vi "Snap.vi"(8 "error in (no error)":errorcluster, 11 "MQTT-Server in":refnum<class "MQTT-Server.lvclass">) -> (0 "error out":errorcluster, 3 "MQTT-Server out":refnum<class "MQTT-Server.lvclass">)   [LabVIEW 2023]
uses:
  MQTT-Server.lvclass
  MQTT-Server.lvclass/MQTT-Server.ctl
  C:/Program Files/National Instruments/LabVIEW 2023/vi.lib/ActorFramework/Actor/Actor.lvclass
  C:/Users/KIV4BP/Documents/Projects/mqtt-budlug/source/MQTT-Server/MQTT-Server/MQTT-Server.lvclass
panel:
  out "Chart":waveform(dbl)[](graph)
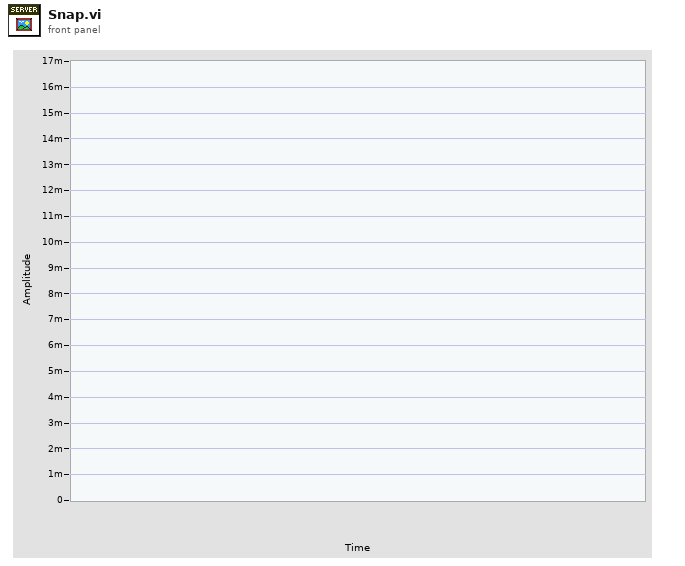
[diagram p1: front panel]
types:
  T1 = typedef "imagedata.ctl" = cluster{"image type":i32, "image depth":i32, "image":u8[], "mask":u8[], "colors":u32[], "Rectangle":cluster{"left":i16, "top":i16, "right":i16, "bottom":i16}}
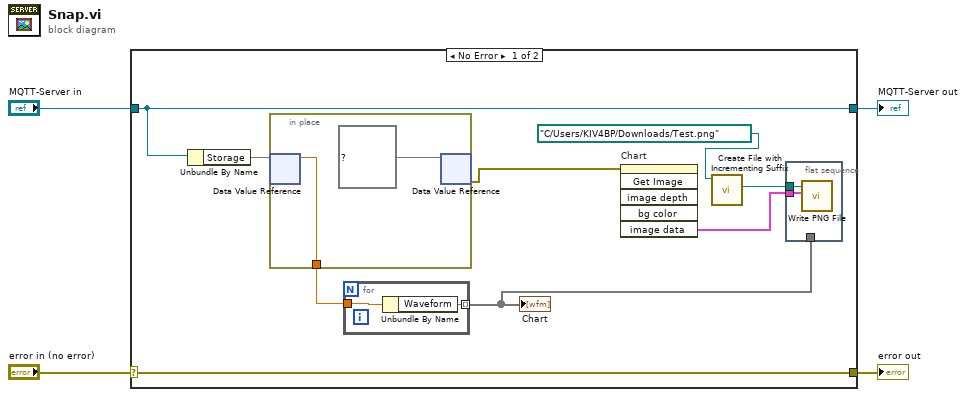
[diagram p0: block diagram]
diagram:
  n1 = case shown="No Error" "error in (no error)" {
    selector: "error in (no error)" -> [w13 w21]
    tunnel: [w13 w21] -> w3
    tunnel: [w12 w20] -> w1
    tunnel: "MQTT-Server in" -> [w12 w20]
    frame No Error {
      n2 = Unbundle By Name(w12) -> ("Storage"=w11)
      n3 = in-place {
        in-place-border: [w18] -> w10
        n4 = in-place-dvr #1(w11) -> (w18:dbl)  [unwired: 1 out]
        n5 = in-place-dvr #1(map{string, waveform(dbl)} {} ("data value")) -> (w8:errorcluster)  [unwired: 1 out]
      }
      n6 = for {
        tunnel: w10 -> [w17]
        tunnel: [w16] -> w5 mode=indexing
        n7 = Unbundle By Name(w17) -> ("Waveform"=w16)
      }
      "Chart" <- w5
      n8 = invoke on="Chart" class="WFChart (strict)" method="Get Image"(error in=w8) -> ("image data"=w9:T1)  [unwired: 5 in, 5 out]
      n9 = call <vilib>:"Create File with Incrementing Suffix.vi"("file path"=path "C:/Users/KIV4BP/Downloads/Test.png" ("path to PNG file")) -> ("actual path"=w6:path)  [unwired: 8 in, 2 out]
      n10 = flat-sequence {
        tunnel: w9 -> [w15]
        tunnel: w6 -> [w14]
        tunnel: w5 -> [_]
        frame #0 {
          n11 = call <vilib>:"Write PNG File.vi"("image data"=w15, "path to PNG file"=w14) -> ()  [unwired: 8 in, 2 out]
        }
      }
    }
    frame Error {
    }
  }
  "error out" <- w3
  "MQTT-Server out" <- w1
